vi "Write Header.vi"(8 "Error In":errorcluster, 11 "Log In":refnum<file>) -> (0 "Error Out":errorcluster, 3 "Log Out":refnum<file>)   [LabVIEW 2015, in "Logger.lvlib" / "File.lvlib"]
uses:
  File.lvlib
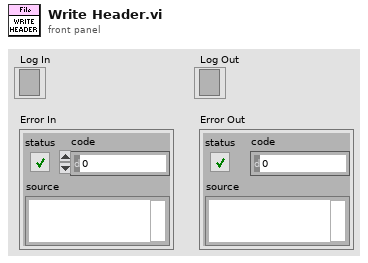
[diagram p1: front panel]
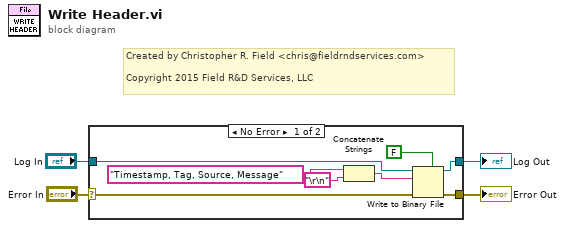
[diagram p0: block diagram]
diagram:
  # "Created by Christopher R. Field <chris@fieldrndservices.com>\n\nCopyright 2015 Field R&D Services, LLC"
  n1 = case shown="No Error" "Error In" {
    selector: "Error In" -> [w9 w13]
    tunnel: "Log In" -> [w11 w14]
    tunnel: [w10 w14] -> w3
    tunnel: [w8 w13] -> w1
    frame No Error {
      n2 = Concatenate Strings("Timestamp, Tag, Source, Message", "\r\n") -> (w6:string)
      n3 = Write to Binary File(file (use dialog)=w11, data=w6, error in=w9, 5:FALSE ("prepend array or string size? (T)")) -> (refnum out=w10:refnum<file>, error out=w8:errorcluster)  [unwired: 2 in, 1 out]
    }
    frame Error {
    }
  }
  "Log Out" <- w3
  "Error Out" <- w1
